vi "MotionProfiles_Init.vi"(4 "Wheel_Diameter (in)":dbl=4.0, 6 "MP_Frame_Rate_(ms)":i32=5, 7 "Encoder_CPR_4x":dbl=240.0, 8 "error in (no error)":errorcluster, 9 "CSV File Path":path=path "/home/lvuser/mp.csv", 10 "PhoenixMotorControlDevRef":T1={"DeviceStatus"={"status"=FALSE, "code"=0, "source"=""}, "Type"=enum."PWM", "PWM"={"PWM Channel"=enum."Invalid", "DeadBand"={"Name"="", "maxPositivePwm"=0, "minPositivePwm"=0, "centerPwm"=0, "maxNegativePwm"=0, "minNegativePwm"=0, "angularRange"=0}}, "CAN"={"Device Number"=0, "SetOutput VI Ref"=variant(refnum<vi> refnum), "GetOutput VI Ref"=variant(refnum<vi> refnum), "Enable VI Ref"=variant(refnum<vi> refnum), "Disable VI Ref"=variant(refnum<vi> refnum), "Data"=variant}, "Invert"=FALSE, "DIO PWM"={"PWM \"Enable\" Channel"=enum."Invalid", "DIOChannel"=enum."Invalid", "PWM Rate"=0.0}}, 11 "MotionProfiles in":refnum<class "MotionProfiles.lvclass">) -> (0 "error out":errorcluster, 1 "Array":i32[](array[numeric]), 3 "MotionProfiles out":refnum<class "MotionProfiles.lvclass">)   [LabVIEW 2017, in "MotionProfiles.lvclass"]
uses:
  MotionProfiles.lvclass
  <vilib>/Rock Robotics/WPI/MotorControl/WPI_MotorControlDeviceRef.ctl
  <vilib>/Rock Robotics/WPI/MotorControl/WPI_MotorControlType.ctl
  <vilib>/Rock Robotics/SystemInterfaces/DIO/FPGA_DIOPWMChannel.ctl
  <vilib>/Rock Robotics/WPI/PWM/WPI_PWMDeadband.ctl
  <vilib>/Rock Robotics/SystemInterfaces/DIO/FPGA_DIOChannel.ctl
  MotionProfile_InternalStateEnum.ctl
  MotionProfile_TalonSetValueEnum.ctl
  MotionProfile_TrajectoryPoint.ctl
  MotionProfiles.lvclass/MotionProfiles.ctl
  <vilib>/Utility/file.llb/Read Delimited Spreadsheet (DBL).vi
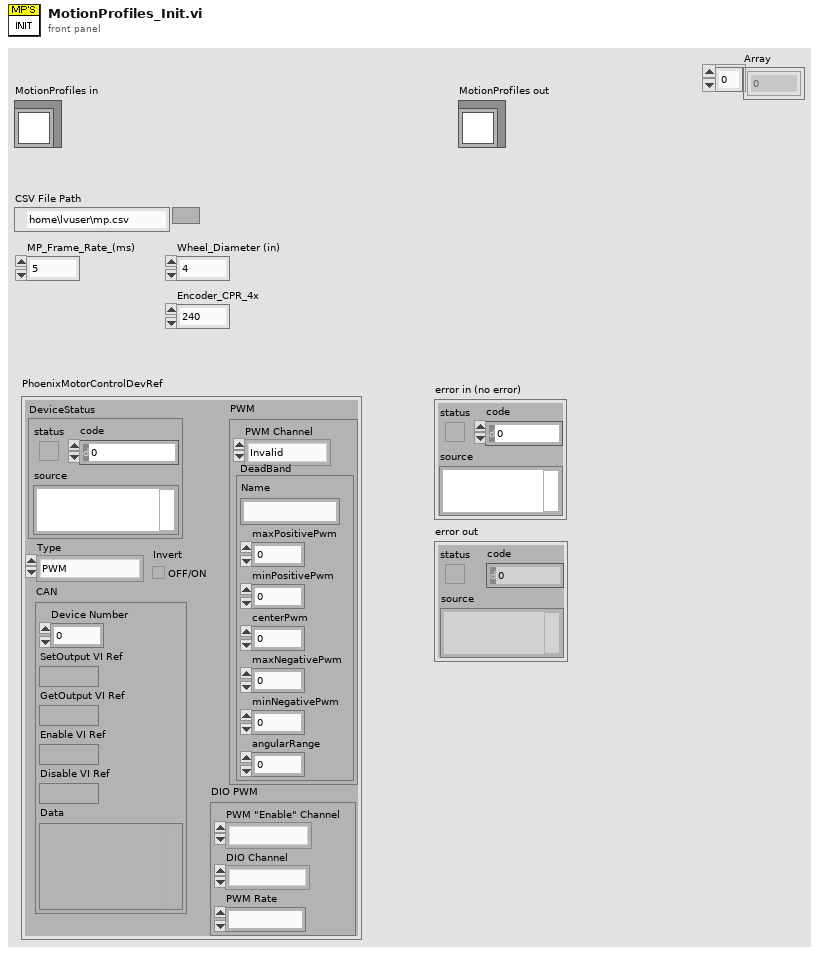
[diagram p1: front panel]
types:
  T1 = typedef "WPI_MotorControlDeviceRef.ctl" = cluster{"DeviceStatus":errorcluster, "Type":T2, "PWM":cluster{"PWM Channel":T3, "DeadBand":T4}, "CAN":cluster{"Device Number":u8, "SetOutput VI Ref":variant, "GetOutput VI Ref":variant, "Enable VI Ref":variant, "Disable VI Ref":variant, "Data":variant}, "Invert":bool, "DIO PWM":cluster{"PWM \"Enable\" Channel":T3, "DIOChannel":T5, "PWM Rate":dbl}}
  T2 = typedef "WPI_MotorControlType.ctl" = enum16{"PWM", "CAN", "DIO PWM"}
  T3 = typedef "FPGA_DIOPWMChannel.ctl" = enum8{"PWM 0", "PWM 1", "PWM 2", "PWM 3", "PWM 4", "PWM 5", "PWM 6", "PWM 7", "PWM 8", "PWM 9", "PWM MXP 0", "PWM MXP 1", "PWM MXP 2", "PWM MXP 3", "PWM MXP 4", "PWM MXP 5", "PWM MXP 6", "PWM MXP 7", "PWM MXP 8", "PWM MXP 9", "Invalid"}
  T4 = typedef "WPI_PWMDeadband.ctl" = cluster{"Name":string, "maxPositivePwm":i32, "minPositivePwm":i32, "centerPwm":i32, "maxNegativePwm":i32, "minNegativePwm":i32, "angularRange":u16}
  T5 = typedef "FPGA_DIOChannel.ctl" = enum8{"DIO 0", "DIO 1", "DIO 2", "DIO 3", "DIO 4", "DIO 5", "DIO 6", "DIO 7", "DIO 8", "DIO 9", "DIO MXP 0", "DIO MXP 1", "DIO MXP 2", "DIO MXP 3", "DIO MXP 4", "DIO MXP 5", "DIO MXP 6", "DIO MXP 7", "DIO MXP 8", "DIO MXP 9", "DIO MXP 10", "DIO MXP 11", "DIO MXP 12", "DIO MXP 13", "DIO MXP 14", "DIO MXP 15", "SPI Port CS1", "SPI Port CS2", "SPI Port CS3", "SPI Port MISO", "SPI Port MOSI", "Invalid"}
  T6 = typedef "MotionProfiles.lvclass/MotionProfile_TrajectoryPoint.ctl" = cluster{"Duration (ms)":u8, "Velocity (u/100ms)":dbl, "Position (units)":dbl, "Profile Slot Select":u8, "Is Last":bool, "Velocity Only":bool, "Zero Position":bool, "Compress Code":u8, "Same Velocity":i32, "Delta Position":i32, "Count":u8, "Invert Motors?":bool}
  T7 = typedef "MotionProfiles.lvclass/MotionProfile_TalonSetValueEnum.ctl" = enum16{"Disable", "Enable", "Hold"}
  T8 = typedef "MotionProfiles.lvclass/MotionProfile_InternalStateEnum.ctl" = enum16{"Nothing", "Send Points to Talon", "Run Profile"}
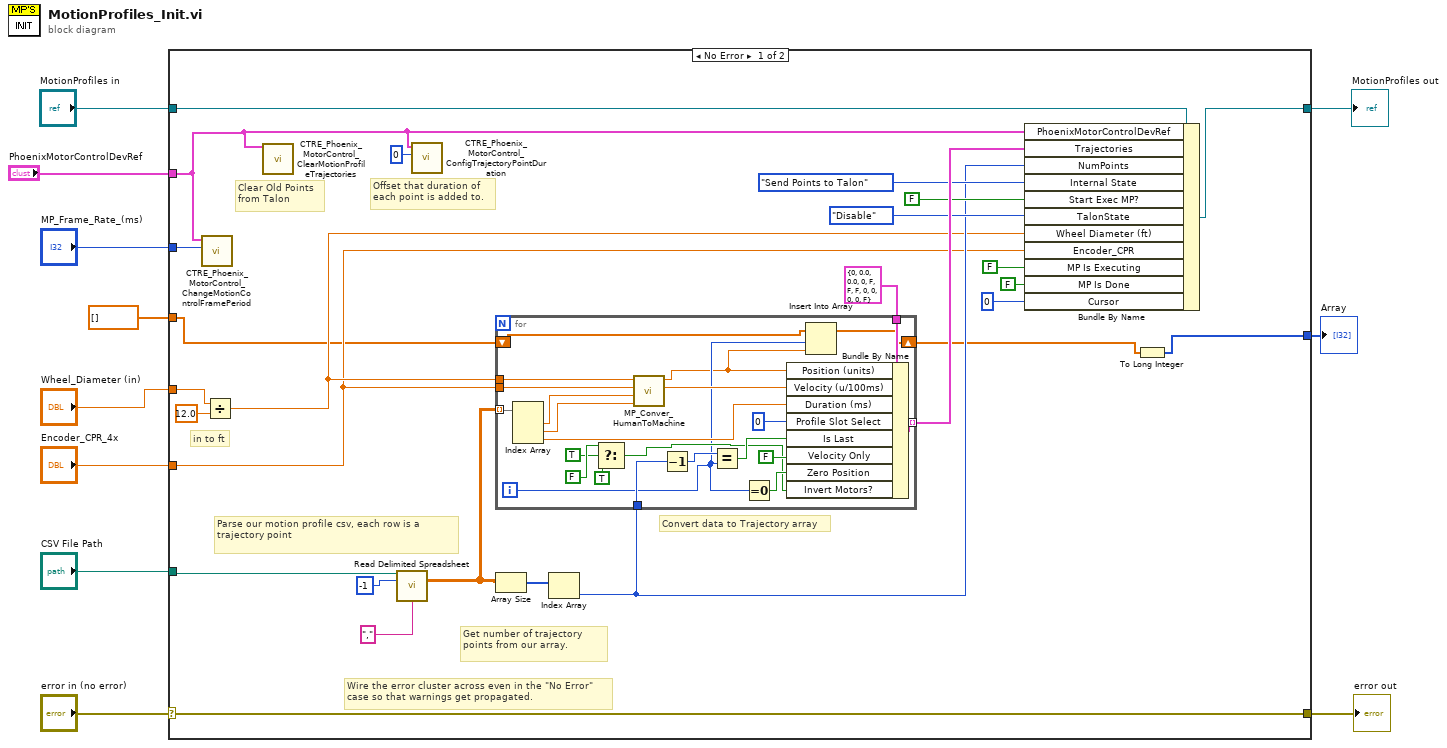
[diagram p0: block diagram]
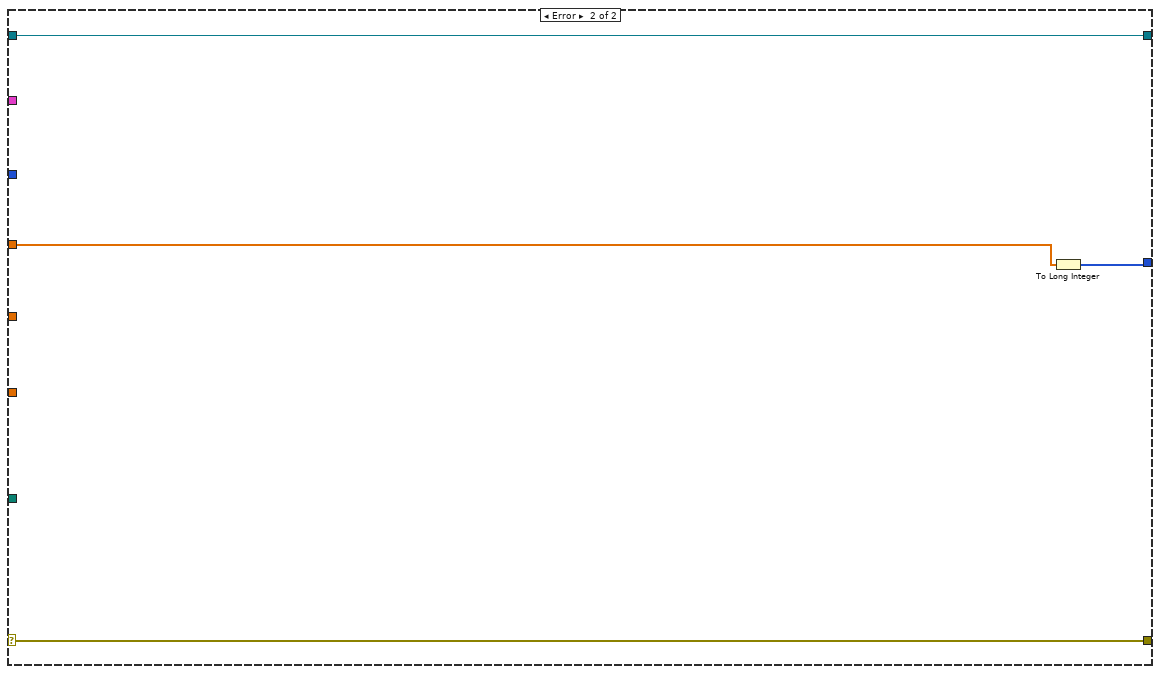
[diagram p2: hidden frame]
diagram:
  n1 = case shown="No Error" "error in (no error)" {
    selector: "error in (no error)" -> [w38 w65]
    tunnel: [w38 w65] -> w10
    tunnel: [w37 w64] -> w8
    tunnel: "MotionProfiles in" -> [w25 w64]
    tunnel: "PhoenixMotorControlDevRef" -> [w20 _]
    tunnel: "CSV File Path" -> [w35 _]
    tunnel: "MP_Frame_Rate_(ms)" -> [w24 _]
    tunnel: "Wheel_Diameter (in)" -> [w30 _]
    tunnel: "Encoder_CPR_4x" -> [w15 _]
    tunnel: dbl[] [] -> [w14 w62]
    tunnel: [w12 w63] -> w1
    frame No Error {
      # "Offset that duration of \neach point is added to."
      # "in to ft"
      # "Clear Old Points\nfrom Talon"
      # "Convert data to Trajectory array"
      # "Get number of trajectory points from our array."
      # "Parse our motion profile csv, each row is a trajectory point"
      # "Wire the error cluster across even in the \"No Error\"\ncase so that warnings get propagated."
      n2 = call <vilib>:"CTRE_Phoenix_MotorControl_ChangeMotionControlFramePeriod.vi"("periodMs"=w24, "PhoenixMotorControlDevRef"=w20) -> ()  [unwired: 8 in, 2 out]
      n3 = Divide(x=w30, y=12.0) -> (x/y=w21:dbl)
      n4 = call <vilib>:"CTRE_Phoenix_MotorControl_ClearMotionProfileTrajectories.vi"("PhoenixMotorControlDevRef"=w20) -> ()  [unwired: 13 in, 2 out]
      n5 = call-poly <vilib>:"Read Delimited Spreadsheet.vi"("file path (dialog if empty)"=w35, "number of rows (all:-1)"=-1, "delimiter (\\t)"="," ("delimiter (\\t)")) -> ("all rows"=w27:dbl[][])  [unwired: 7 in, 5 out]
      n6 = call <vilib>:"CTRE_Phoenix_MotorControl_ConfigTrajectoryPointDuration.vi"("durationMs"=0, "PhoenixMotorControlDevRef"=w20) -> ()  [unwired: 8 in, 2 out]
      n7 = Array Size(array=w27) -> (size(s)=w26:i32[])
      n8 = Index Array(array=w26) -> (element=w22:i32)  [unwired: 1 in]
      n9 = for {
        tunnel: [w59] -> w34 mode=indexing
        tunnel: w27 -> [w57] mode=indexing
        tunnel: T6 {"Duration (ms)"=0, "Velocity (u/100ms)"=0.0, "Position (units)"=0.0, "Profile Slot Select"=0, "Is Last"=FALSE, "Velocity Only"=FALSE, "Zero Position"=FALSE, "Compress Code"=0, "Same Velocity"=0, "Delta Position"=0, "Count"=0, "Invert Motors?"=FALSE} ("Motion Profile Trajectory Point") -> [w56]
        tunnel: w22 -> [w52]
        tunnel: w21 -> [w51]
        tunnel: w15 -> [w50]
        shift-right: [w42] -> w13
        shift-left: w14 -> [w44]
        i -> [w41]
        n10 = Index Array(array=w57) -> (element #1=w49:dbl, element #2=w48:dbl, element #3=w55:dbl)  [unwired: 3 in]
        n11 = Select(t=FALSE, s=TRUE, f=TRUE) -> (s? t:f=w45:bool)
        n12 = call "MP_Conver_HumanToMachine.vi"("Vel_In (ft/s)"=w48, "Pos_In (ft)"=w49, "CPR"=w50, "Diameter (ft)"=w51) -> ("Vel_Out (u/100ms)"=w43:dbl, "Pos_Out (u)"=w40:dbl)  [unwired: 4 in]
        n13 = Decrement(x=w52) -> (x-1=w53:i32)
        n14 = Equal?(x=w53, y=w41) -> (x = y?=w54:bool)
        n15 = Equal To 0?(x=w41) -> (x = 0?=w60:bool)
        n16 = Bundle By Name(cluster=w56, "Position (units)"=w40, "Velocity (u/100ms)"=w43, "Duration (ms)"=w55, "Profile Slot Select"=u8 0, "Is Last"=w54, "Velocity Only"=FALSE, "Zero Position"=w60, "Invert Motors?"=w45) -> (w59:T6)
        n17 = Insert Into Array(array=w44, index=w41, new element=w40) -> (w42:dbl[])
      }
      n18 = Bundle By Name(cluster=w25, "PhoenixMotorControlDevRef"=w20, "Trajectories"=w34, "NumPoints"=w22, "Internal State"=MotionProfile_InternalStateEnum."Send Points to Talon", "Start Exec MP?"=FALSE, "TalonState"=MotionProfile_TalonSetValueEnum."Disable" ("TalonSetValue"), "Wheel Diameter (ft)"=w21, "Encoder_CPR"=w15, "MP Is Executing"=FALSE, "MP Is Done"=FALSE, "Cursor"=u32 0) -> (w37:refnum<class "MotionProfiles.lvclass">)
      n19 = To Long Integer(number=w13) -> (32bit integer=w12:i32[])
    }
    frame Error {
      n20 = To Long Integer(number=w62) -> (32bit integer=w63:i32[])
    }
  }
  "error out" <- w10
  "MotionProfiles out" <- w8
  "Array" <- w1
